vi "MethodGuide.vi"(1 "Attributes":string[](array[string])) -> (15 "Preview":string, 16 "Canceled":bool)   [LabVIEW 2020, in "VINode.lvclass"]
uses:
  <resource>/Framework/Providers/Open_GDS/UML/VINode_class/VINode.lvclass
  <resource>/Framework/Providers/Open_GDS/ClassProviders/Common/CommonVIs/CommonVIs_VisibilityType.ctl
  <resource>/Framework/Providers/Open_GDS/UML/VINode_class/EventType.ctl
  <resource>/Framework/Providers/Open_GDS/UML/ContextHelp/ContextHelp_HelpTexts.ctl
panel:
  in  "Type":T1
  in  "Help":bool
  in  "Cancel":bool
  in  "OK":bool
  in  "Visibility":T2
  in  "Event Name":string(combo)
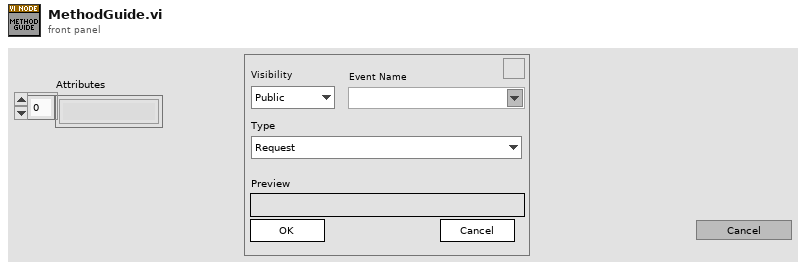
[diagram p1: front panel]
types:
  T1 = typedef "EventType.ctl" = enum16{"Request", "Request and Wait For Reply", "Roundtrip", "Broadcast"}
  T2 = typedef "CommonVIs_VisibilityType.ctl" = enum16{"Public", "Private", "Protected"}
  T3 = typedef "ContextHelp_HelpTexts.ctl" = enum16{"None(Hide)", "Default", "Help", "Welcome", "GettingStarted", "ClassDiagram_Help", "SequenceDiagram_Help", "UseCaseDiagram_Help", "BSelect", "BClass", "BInterface", "BPackage", "BNote", "BDependency", "BInheritance", "BInterfaceImplementation", "BAssociation", "BAggregation", "BCompAggregation", "BNoteConnector", "BObject", "BActionBar", "BCall", "BSystem", "BActor", "BUseCase", "BGeneralization", "BIncludes", "BExtends", "BUseCaseDiagramAssociation", "ClassRelationshipEdge editDialog_Bent Style", "ClassRelationshipEdge editDialog_RelationType", "ClassRelationshipEdge editDialog_Reverse association", "ClassRelationshipEdge editDialog_Start label", "ClassRelationshipEdge editDialog_Middle label", "ClassRelationshipEdge editDialog_End label", "UMLEditor reversedEngineering_Pathes", "ReversedEngineering StateReverseDialog_Help", "ReversedEngineering StateQueuedSettings_Help", "UMLEditor reversedEngineering_AddTopVIs", "UMLEditor reversedEngineering_AddClasses", "UMLEditor reversedEngineering_AddDirs", "UMLEditor reversedEngineering_Recursively", "UMLEditor reversedEngineering_Remove", "UMLEditor reversedEngineering_ClearList", "UMLEditor reversedEngineering_HideSubAss", "UMLEditor reversedEngineering_CreateTypes", "UMLEditor reversedEngineering_OnlyInheritance", "UMLEditor reversedEngineering_CreateApplication", "UMLEditor reversedEngineering_OK", "UMLEditor reversedEngineering_Cancel", "UMLEditor reversedEngineering_Help", "UMLEditor createWizardScriptFile_ScriptfilePath", "UMLEditor createWizardScriptFile_ClassPath", "UMLEditor createWizardScriptFile_Use", "UMLEditor createWizardScriptFile_PrivateDirName", "UMLEditor createWizardScriptFile_DirAppend", "UMLEditor createWizardScriptFile_Separator Character", "UMLEditor createWizardScriptFile_OK", "UMLEditor createWizardScriptFile_Cancel", "UMLEditor createWizardScriptFile_Help", "ClassNode editDialog_Class Name", "InterfaceNode editDialog_Class Name", "ClassNode editDialog_Attribute", "ClassNode editDialog_Methods", "InterfaceNode editDialog_Methods", "ClassNode editDialog_connection", "InterfaceNode editDialog_connection", "ClassNode editDialog_StereoType", "ClassNode editDialog_ShowAttrib", "ClassNode editDialog_ShowMethods", "ClassNode editDialog_ClassPath", "ClassNode editDialog_AddAttribute", "ClassNode editDialog_AddMethod", "InterfaceNode editDialog_AddMethod", "ClassNode AttributeGuide_AttributeName", "ClassNode AttributeGuide_Array?", "ClassNode AttributeGuide_Data Type", "ClassNode AttributeGuide_RefName", "ClassNode AttributeGuide_Preview", "ClassNode AttributeGuide_OK", "ClassNode AttributeGuide_Cancel", "ClassNode MethodGuide_Visibility", "ClassNode MethodGuide_Method Name", "ClassNode MethodGuide_Preview", "ClassNode MethodGuide_OK", "ClassNode MethodGuide_Cancel", "CallNode EditCallProperties_AllButtons", "ObjectNode EditObjectlProperties_AllButtons", "ActorNode EditActorProperties_AllButtons", "UseCaseRelationshipNode EditUseCaselProperties_AllButtons", "UseCaseNode EditUseCaselProperties_AllButtons", "SystemNode EditSystemProperties_AllButtons", "ReversedEngineering UpdateAttributes_AllButtons", "StateNode editDialog_AllButtons", "StateTransition editDialog_AllButtons", "ArrangeNodes Main_Picture", "ArrangeNodes Main_Zoom", "ArrangeNodes Main_Auto Zoom", "ArrangeNodes Main_shorten", "ArrangeNodes Main_Min Length", "ArrangeNodes Main_Max Length", "ArrangeNodes Main_increase", "ArrangeNodes Main_decrease", "ArrangeNodes Main_Shake", "ArrangeNodes Main", "BState", "BInitialState", "BFinalState", "BStateTransition", "StateDiagram_Help", "StateDiagram_PropertiesAllButtons", "ReversedEngineering StateReverseDialog_ClearStates", "ReversedEngineering StateReverseDialog_UseQueuedStateMachines", "ReversedEngineering StateReverseDialog_QueuedSettings", "ReversedEngineering StateReverseDialog_SearchForVIs", "ReversedEngineering StateReverseDialog_SearchCriteria", "OptionsDialog_ClassBasePath", "OptionsDialog_VIPath", "OptionsDialog_ApplicationPath", "OptionsDialog_WizDir", "OptionsDialog_IniFilePath", "OptionsDialog_DefineColors", "OptionsDialog_Help", "OptionsDialog_CreateTypes", "ClassRelationshipEdge editDialog_SplitWire"}
  T4 = typedef "ContextHelp_ShowType.ctl" = cluster{"Header":string, "Picture":picture, "Text":string}
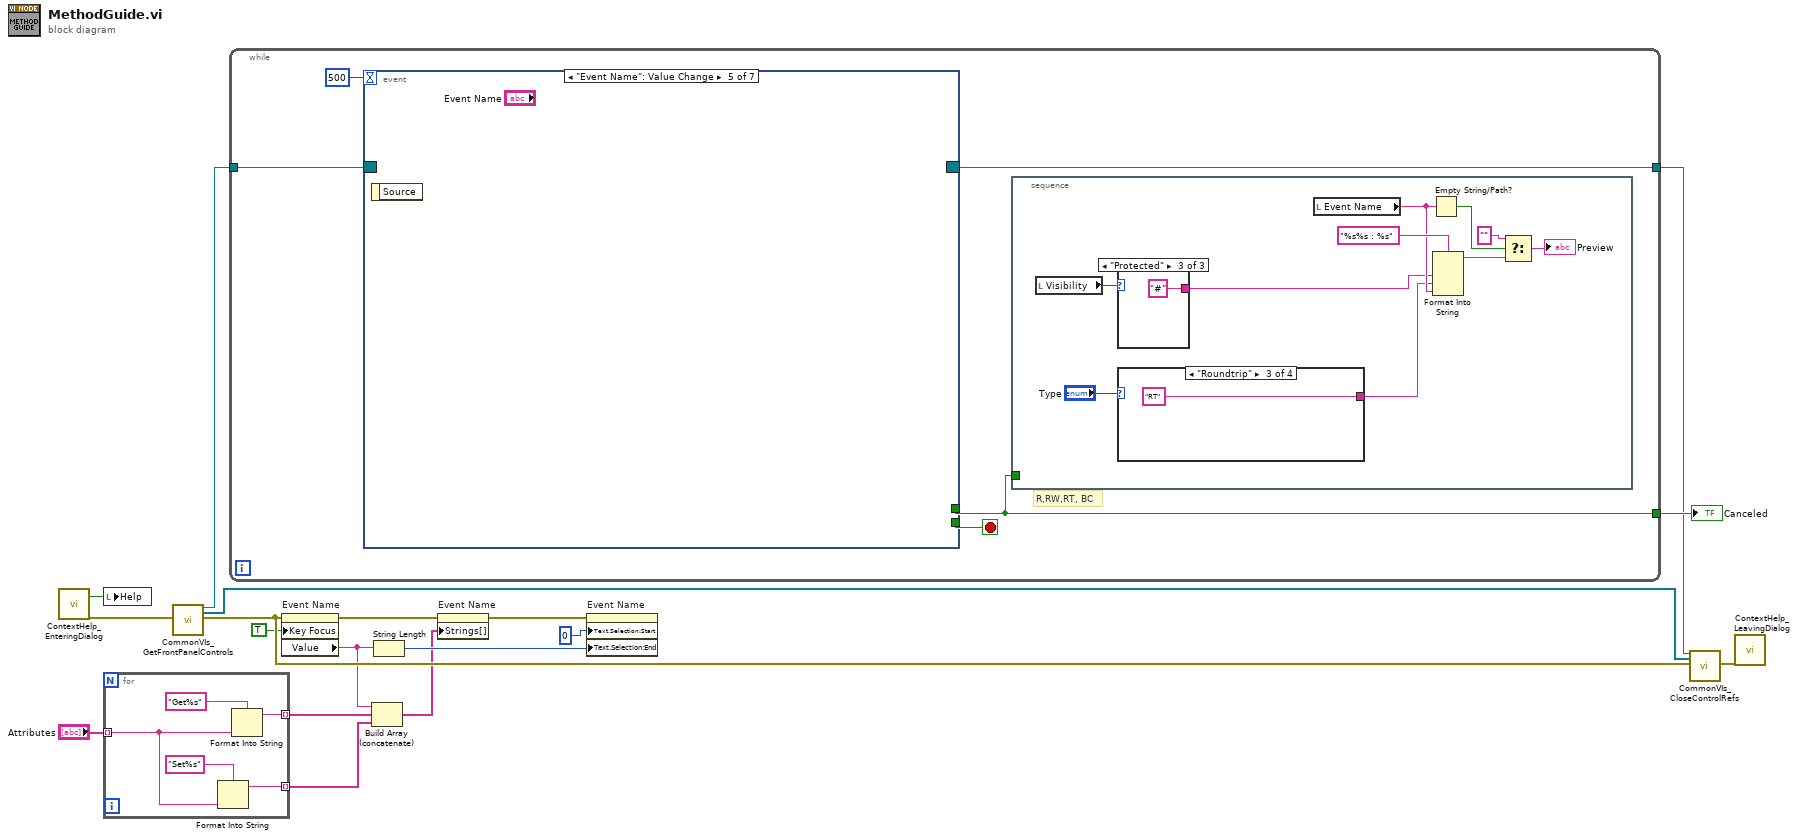
[diagram p0: block diagram]
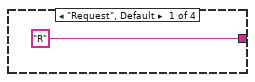
[diagram p2: hidden frame]
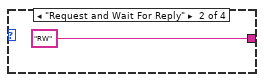
[diagram p3: hidden frame]
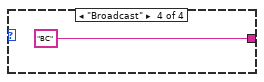
[diagram p4: hidden frame]
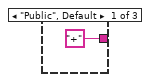
[diagram p5: hidden frame]
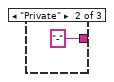
[diagram p6: hidden frame]
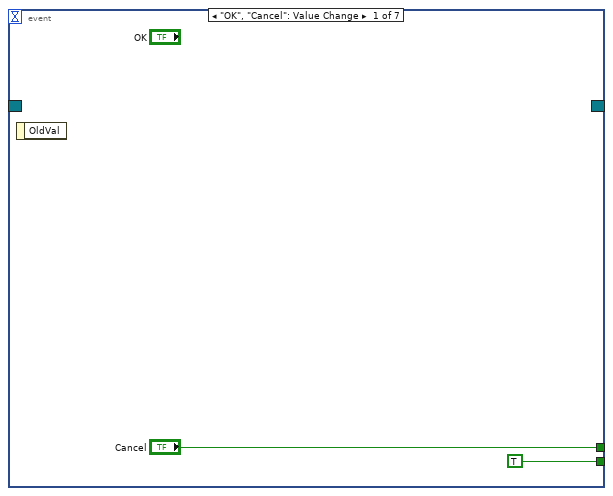
[diagram p7: hidden frame]
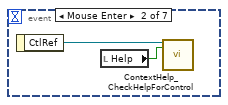
[diagram p8: hidden frame]
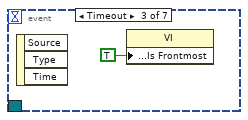
[diagram p9: hidden frame]
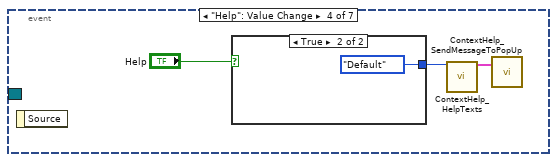
[diagram p10: hidden frame]
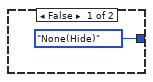
[diagram p11: hidden frame]
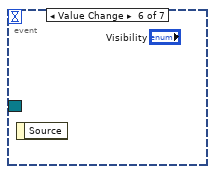
[diagram p12: hidden frame]
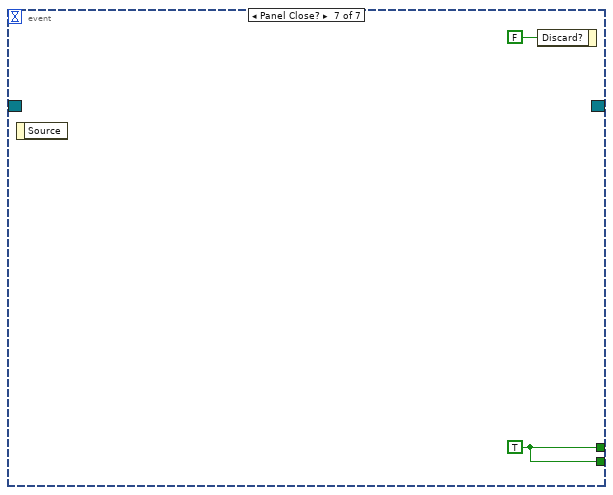
[diagram p13: hidden frame]
diagram:
  n1 = call <resource>:"ContextHelp_EnteringDialog.vi"() -> ("HelpStatus"=w17:bool, "error out"=w15:errorcluster)  [unwired: 3 in, 15 out]
  n2 = local write "Help"(w17) -> ()
  n3 = for {
    tunnel: [w20] -> w3 mode=indexing
    tunnel: "Attributes" -> [w21] mode=indexing
    tunnel: [w19] -> w1 mode=indexing
    n4 = Format Into String(format string="Set%s", w21) -> (resulting string=w19:string)  [unwired: 2 in, 1 out]
    n5 = Format Into String(format string="Get%s", w21) -> (resulting string=w20:string)  [unwired: 2 in, 1 out]
  }
  n6 = call <resource>:"CommonVIs_GetFrontPanelControls.vi"("error in (no error)"=w15) -> ("Event Registration Refnum"=w13:refnum<event-registration>, "ControlRefs"=w16:refnum<vi>[], "error out"=w11:errorcluster)  [unwired: 1 in, 15 out]
  n7 = while {
    tunnel: [w24] -> w18
    tunnel: w13 -> [w27]
    tunnel: [w26] -> w12
    stop <- w28 stop-if-true
    # "R,RW,RT, BC"
    n8 = event shown="[4] \"Event Name\": Value Change" {
      selector: w27 -> [_ _ _ _ _ _ _]
      dyn-events: [_ _ _ _ _ _ _] -> w26
      timeout: 500 -> [_ _ _ _ _ _ _]
      tunnel: ["Cancel" _ _ _ _ _ w56] -> w24
      tunnel: [TRUE _ _ _ _ _ w56] -> w28
      event "OK", "Cancel": Value Change {
        n9 = event-data() -> ()  [unwired: 2 out]
      }
      event Mouse Enter {
        n10 = event-data() -> ("CtlRef"=w48:refnum<vi>)  [unwired: 1 out]
        n11 = local read "Help"() -> (w49:bool)
        n12 = call <resource>:"ContextHelp_CheckHelpForControl.vi"("Ctl Refnum"=w48, "Help"=w49) -> ()  [unwired: 1 in, 17 out]
      }
      event Timeout {
        n13 = event-data() -> ()  [unwired: 4 out]
        n14 = property class="VI"("Front Panel Window:Is Frontmost"=TRUE) -> ()  [unwired: 2 in, 2 out]
      }
      event "Help": Value Change {
        n15 = event-data() -> ()  [unwired: 2 out]
        n16 = case shown="True" "Help" {
          tunnel: [ContextHelp_HelpTexts."None(Hide)" ("HelpText") ContextHelp_HelpTexts."Default" ("HelpText")] -> w52
          frame False {
          }
          frame True {
          }
        }
        n17 = call <resource>:"ContextHelp_HelpTexts.vi"("HelpText (enum or string)"=w52) -> ("HelpOut"=w53:T4)  [unwired: 18 out]
        n18 = call <resource>:"ContextHelp_SendMessageToPopUp.vi"("PopUpMessage"=w53) -> ()  [unwired: 2 in, 17 out]
      }
      event "Event Name": Value Change {
        n19 = event-data() -> ()  [unwired: 2 out]
      }
      event Value Change {
        n20 = event-data() -> ()  [unwired: 2 out]
      }
      event Panel Close? {
        w56 = TRUE ("Discard?")
        n21 = event-data() -> ()  [unwired: 2 out]
        n22 = event-data("Discard?"=FALSE) -> ()  [unwired: 1 in, 1 out]
      }
    }
    n23 = stacked-sequence {
      tunnel: w24 -> [_]
      frame #0 {
        n24 = local read "Visibility"() -> (w37:T2)
        n25 = case shown="\"Protected\"" w37 {
          tunnel: ["+" "-" "#"] -> w31
          frame "Public", Default {
          }
          frame "Private" {
          }
          frame "Protected" {
          }
        }
        n26 = case shown="\"Roundtrip\"" "Type" {
          tunnel: ["R" "RW" "RT" "BC"] -> w29
          frame "Request", Default {
          }
          frame "Request and Wait For Reply" {
          }
          frame "Roundtrip" {
          }
          frame "Broadcast" {
          }
        }
        n27 = local read "Event Name"() -> (w32:string)
        n28 = Empty String/Path?(string/path=w32) -> (empty?=w36:bool)
        n29 = Format Into String(format string="%s%s : %s", w31, w29, w32) -> (resulting string=w35:string)  [unwired: 2 in, 1 out]
        n30 = Select(t="", s=w36, f=w35) -> (s? t:f=→"Preview":string)
      }
    }
  }
  "Canceled" <- w18
  n31 = property on="Event Name" class="CmbBox"(error in=w11, "Key Focus"=TRUE ("Front Panel Window:Is Frontmost")) -> (error out=w7:errorcluster, "Value"=w5:string)  [unwired: 1 in, 1 out]
  n32 = Build Array (concatenate)(w5, w3, w1) -> (w4:string[])
  n33 = String Length(string=w5) -> (length=w8:i32)
  n34 = property on="Event Name" class="CmbBox"(error in=w7, "Strings[]"=w4) -> (error out=w6:errorcluster)  [unwired: 1 in, 1 out]
  n35 = property on="Event Name" class="CmbBox"(error in=w6, "Text.Selection:Start"=u32 0, "Text.Selection:End"=w8) -> ()  [unwired: 1 in, 2 out]
  n36 = call <resource>:"CommonVIs_CloseControlRefs.vi"("Event Registration Refnum"=w12, "ControlRefs"=w16, "error in (no error)"=w11) -> ("error out"=w14:errorcluster)  [unwired: 16 out]
  n37 = call <resource>:"ContextHelp_LeavingDialog.vi"("error in (no error)"=w14) -> ()  [unwired: 2 in, 17 out]
